vi "Auto_guider.vi"() -> ()   [LabVIEW 2018]
uses:
  Global_Telescopio.vi
panel:
  in  "Case Constant\n(See Context Help) 2":bool
  in  "Case Constant\n(See Context Help)":bool=TRUE
  out "substring 3":string
  out "substring 2":string
  out "concatenated string":string
  out "substring":string
  out "result string":string
  in  "esc_placa":string="0.462"
  out "Serial Settings:Number of Bytes at Serial Port":u32
  in  "guide_esp":string="S"
  in  "guide_cas":string="S"
  in  "guide_str":string="04/10/09  1:18:34\u000013 27 13\u0000-12 45 20\u0000"
  in  "guide_ang":string=" 281.52"
  in  "guide_nor":string="  11.53"
  in  "Tx_sts":u8[](array[numeric])=[22, 2, 1, 0, 83, 0, 0]
  out "rxsts 3":bool
  in  "SYN | ETX":u8[](array[numeric])=[22, 3] format="%02.0f"
  in  "tel_sts2":u8[](array[numeric])=[0, 0, 0] format="%02.0f"
  in  "Tx_ena":u8[](array[numeric])=[22, 2, 1, 0, 72, 0, 0] format="%02.0f"
  out "tel_sts1":bool[](array[boolean])=[TRUE, TRUE, TRUE, TRUE, FALSE, FALSE, TRUE]
  out "guide_dec":dbl format="%07.2g"
  out "guide_dir_ns":string
  out "guide_asc":dbl format="%07.2g"
  out "guide_dir_we":string
  in  "SYN | ACK":u8[](array[numeric])=[22, 6] format="%02.0f"
  out "rxsts":bool
  in  "Tx_nak":u8[](array[numeric])=[22, 21]
  out "Data rx guider":string
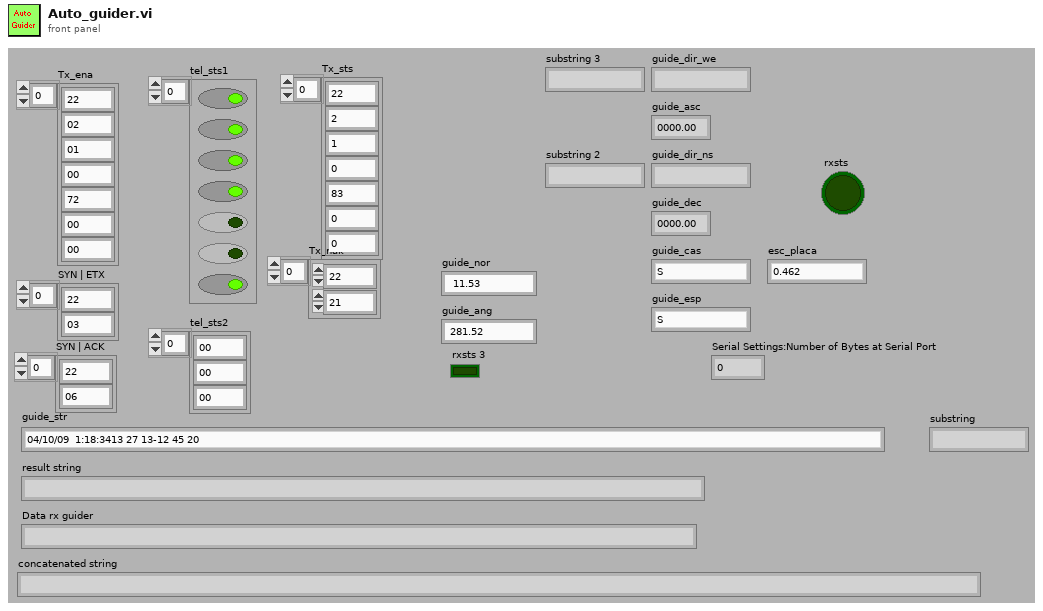
[diagram p1: front panel]
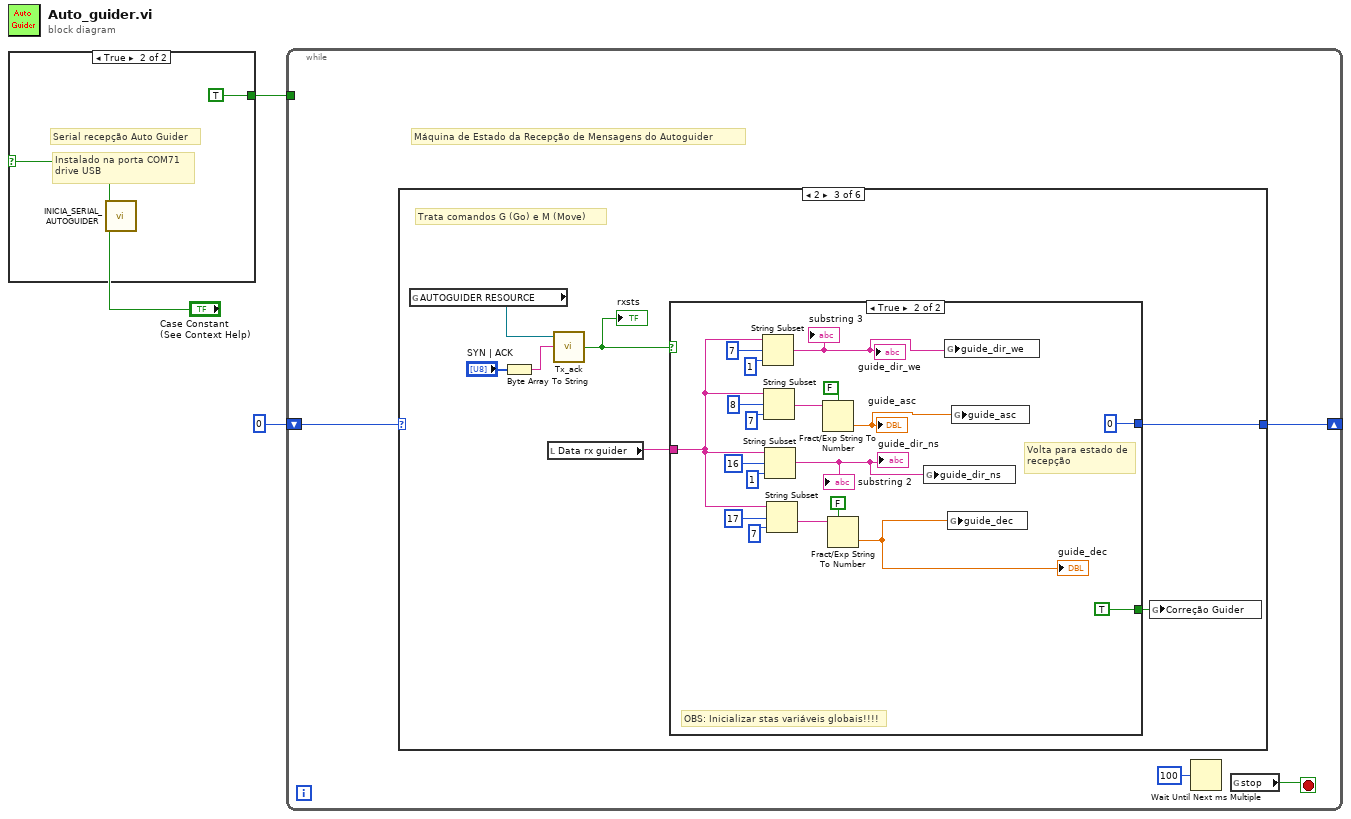
[diagram p0: block diagram]
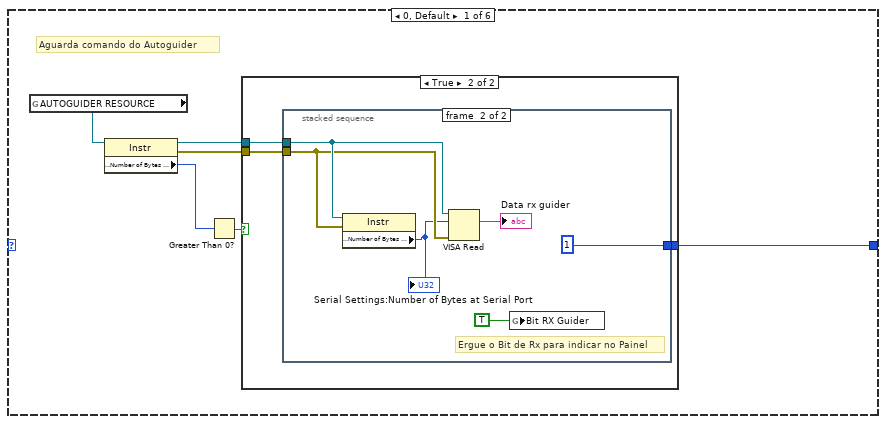
[diagram p3: hidden frame]
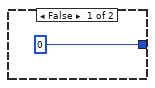
[diagram p4: hidden frame]
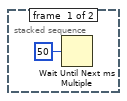
[diagram p5: hidden frame]
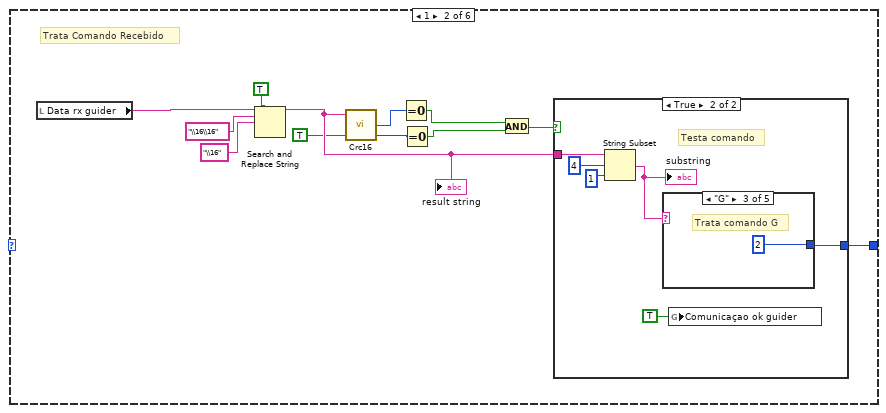
[diagram p6: hidden frame]
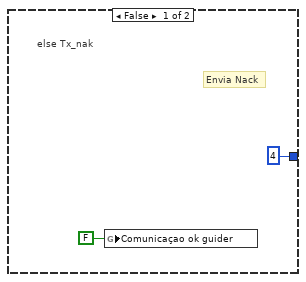
[diagram p7: hidden frame]
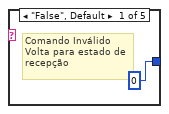
[diagram p8: hidden frame]
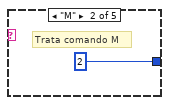
[diagram p9: hidden frame]
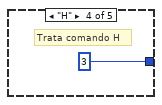
[diagram p10: hidden frame]
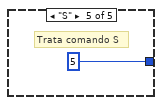
[diagram p11: hidden frame]
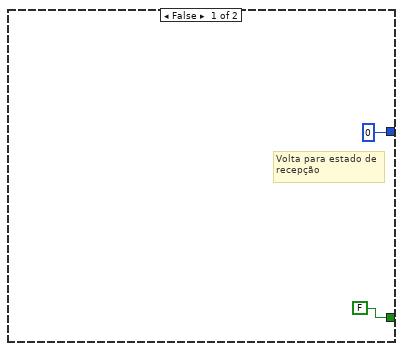
[diagram p12: hidden frame]
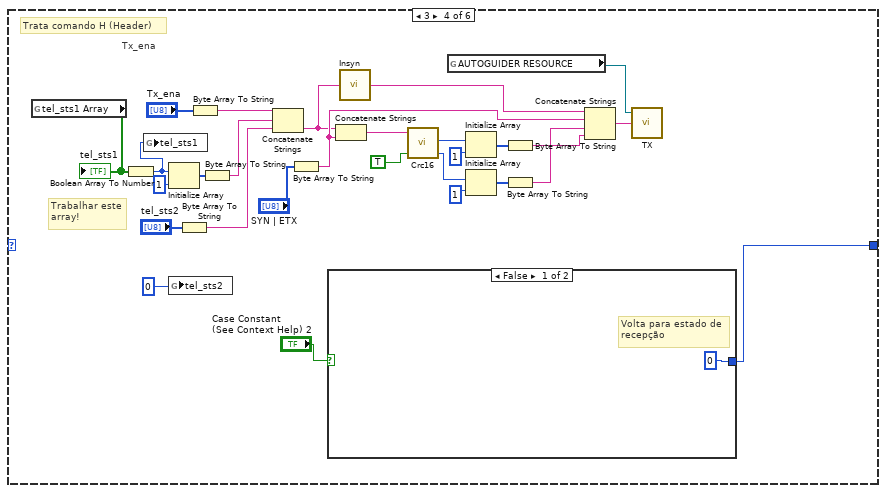
[diagram p13: hidden frame]
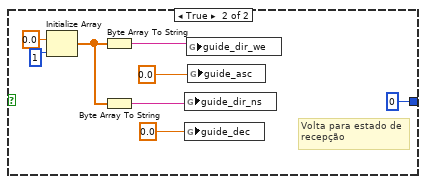
[diagram p14: hidden frame]
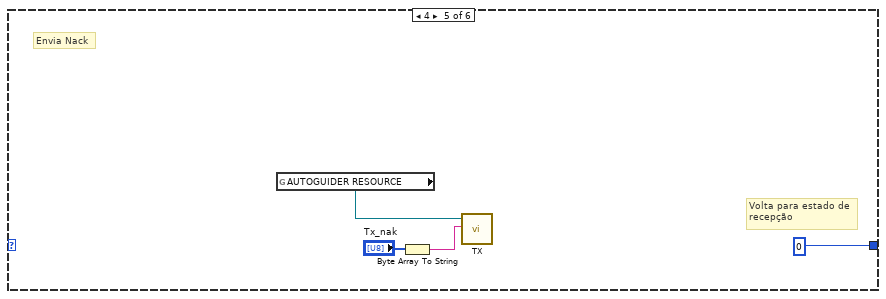
[diagram p15: hidden frame]
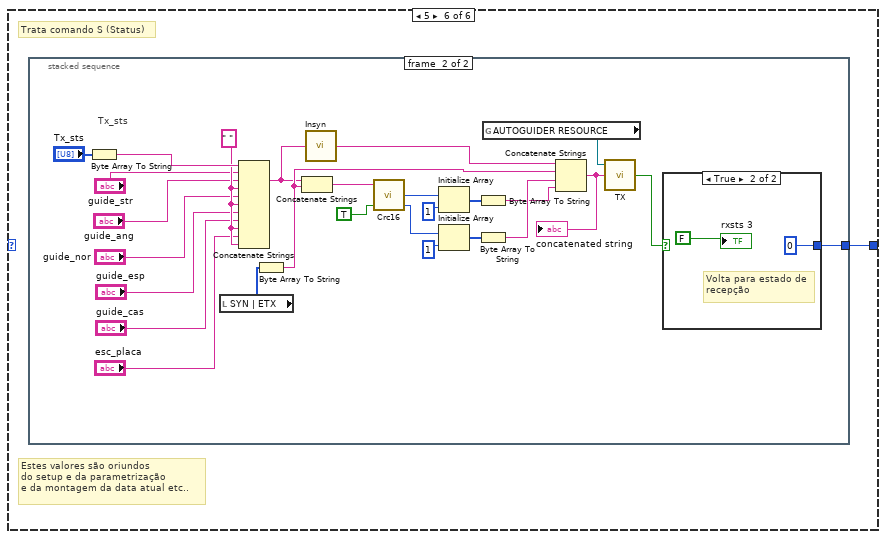
[diagram p16: hidden frame]
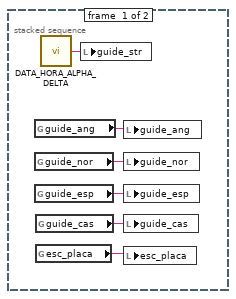
[diagram p17: hidden frame]
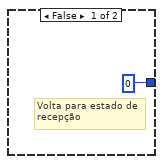
[diagram p18: hidden frame]
diagram:
  n1 = case shown="True" "Case Constant\n(See Context Help)" {
    tunnel: [_ TRUE] -> w1
    frame False {
    }
    frame True {
      # "Instalado na porta COM71\ndrive USB"
      # "Serial recepção Auto Guider"
      n2 = call "INICIA_SERIAL_AUTOGUIDER.vi"() -> ()  [unwired: 6 in, 1 out]
    }
  }
  n3 = while {
    shift-right: [w5] -> _
    shift-left: 0 -> [w6]
    tunnel: w1 -> [_]
    stop <- w8 stop-if-true
    # "Máquina de Estado da Recepção de Mensagens do Autoguider"
    n4 = case shown="2" w6 {
      tunnel: [w9 w37 w52 w83 0 w120] -> w5
      frame 0, Default {
        # "Aguarda comando do Autoguider"
        n5 = global read "Global_Telescopio.vi" "AUTOGUIDER RESOURCE"() -> (w11:refnum<visa-resource-name>)
        n6 = property class="Instr"(reference=w11) -> (reference out=w14:refnum<visa-resource-name>, error out=w13:errorcluster, "Serial Settings:Number of Bytes at Serial Port"=w12:u32)  [unwired: 1 in]
        n7 = Greater Than 0?(x=w12) -> (x > 0?=w10:bool)
        n8 = case shown="True" w10 {
          tunnel: w14 -> [_ w18]
          tunnel: w13 -> [_ w17]
          tunnel: [0 w16] -> w9
          frame False {
          }
          frame True {
            n9 = stacked-sequence {
              tunnel: w18 -> [_ w25]
              tunnel: w17 -> [_ w24]
              tunnel: [_ 1] -> w16
              frame #0 {
                n10 = Wait Until Next ms Multiple(millisecond multiple=u32 50) -> ()  [unwired: 1 out]
              }
              frame #1 {
                # "Ergue o Bit de Rx para indicar no Painel"
                n11 = property class="Instr"(reference=w25, error in=w24) -> ("Serial Settings:Number of Bytes at Serial Port"=w23:u32)  [unwired: 2 out]
                "Serial Settings:Number of Bytes at Serial Port" <- w23
                n12 = VISA Read(VISA resource name=w25, byte count=w23, error in (no error)=w24) -> (read buffer=→"Data rx guider":string)  [unwired: 3 out]
                n13 = global write "Global_Telescopio.vi" "Bit RX Guider"(TRUE) -> ()
              }
            }
          }
        }
      }
      frame 1 {
        # "Trata Comando Recebido"
        n14 = local read "Data rx guider"() -> (w33:string)
        n15 = Search and Replace String(replace all?=TRUE ("replace all? (F)"), input string=w33, search string="\\16\\16", replace string="\\16" ("replace string (\"\")")) -> (result string=w32:string)  [unwired: 4 in, 3 out]
        "result string" <- w32
        n16 = call "Crc16.vi"("Habilita"=TRUE, "tx_rx_buf"=w32) -> ("crc_lo"=w29:u8, "crc_hi"=w30:u8)  [unwired: 1 in, 1 out]
        n17 = Equal To 0?(x=w30) -> (x = 0?=w26:bool)
        n18 = Equal To 0?(x=w29) -> (x = 0?=w27:bool)
        n19 = And(x=w26, y=w27) -> (x .and. y?=w28:bool)
        n20 = case shown="True" w28 {
          tunnel: [4 w45] -> w37
          tunnel: w32 -> [_ w44]
          frame False {
            # "else Tx_nak"
            # "Envia Nack"
            n21 = global write "Global_Telescopio.vi" "Comunicaçao ok guider"(FALSE ("Comunicaçao ok guider")) -> ()
          }
          frame True {
            # "Testa comando"
            n22 = String Subset(string=w44, offset (0)=4, length (rest)=1 ("length (rest)")) -> (substring=w41:string)
            "substring" <- w41
            n23 = case shown="\"G\"" w41 {
              tunnel: [0 2 2 3 5] -> w45
              frame "False", Default {
                # "Comando Inválido\nVolta para estado de\nrecepção"
              }
              frame "M" {
                # "Trata comando M"
              }
              frame "G" {
                # "Trata comando G"
              }
              frame "H" {
                # "Trata comando H"
              }
              frame "S" {
                # "Trata comando S"
              }
            }
            n24 = global write "Global_Telescopio.vi" "Comunicaçao ok guider"(TRUE ("Comunicaçao ok guider")) -> ()
          }
        }
      }
      frame 2 {
        # "Trata comandos G (Go) e M (Move)"
        n25 = global read "Global_Telescopio.vi" "AUTOGUIDER RESOURCE"() -> (w54:refnum<visa-resource-name>)
        n26 = Byte Array To String(unsigned byte array="SYN | ACK") -> (string=w55:string)
        n27 = local read "Data rx guider"() -> (w53:string)
        n28 = call "Tx_ack.vi"("txbuf"=w55, "VISA resource name"=w54) -> ("envio OK"=w57:bool)  [unwired: 1 in, 2 out]
        "rxsts" <- w57
        n29 = case shown="True" w57 {
          tunnel: w53 -> [_ w74]
          tunnel: [0 0] -> w52
          tunnel: [FALSE ("Correção Guider") TRUE ("Correção Guider")] -> w51
          frame False {
            # "Volta para estado de\nrecepção"
          }
          frame True {
            # "OBS: Inicializar stas variáveis globais!!!!"
            # "Volta para estado de\nrecepção"
            n30 = String Subset(string=w74, offset (0)=7, length (rest)=1 ("length (rest)")) -> (substring=w64:string)
            "guide_dir_we" <- w64
            "substring 3" <- w64
            n31 = String Subset(string=w74, offset (0)=8, length (rest)=7 ("length (rest)")) -> (substring=w68:string)
            n32 = String Subset(string=w74, offset (0)=16, length (rest)=1 ("length (rest)")) -> (substring=w62:string)
            "guide_dir_ns" <- w62
            "substring 2" <- w62
            n33 = String Subset(string=w74, offset (0)=17, length (rest)=7 ("length (rest)")) -> (substring=w67:string)
            n34 = Fract/Exp String To Number(use system decimal point (T)=FALSE, string=w68) -> (number=w63:dbl)  [unwired: 2 in, 1 out]
            "guide_asc" <- w63
            n35 = Fract/Exp String To Number(use system decimal point (T)=FALSE, string=w67) -> (number=w61:dbl)  [unwired: 2 in, 1 out]
            "guide_dec" <- w61
            n36 = global write "Global_Telescopio.vi" "guide_dir_ns"(w62) -> ()
            n37 = global write "Global_Telescopio.vi" "guide_dir_we"(w64) -> ()
            n38 = global write "Global_Telescopio.vi" "guide_dec"(w61) -> ()
            n39 = global write "Global_Telescopio.vi" "guide_asc"(w63) -> ()
          }
        }
        n40 = global write "Global_Telescopio.vi" "Correção Guider"(w51) -> ()
      }
      frame 3 {
        # "Trabalhar este\narray!"
        # "Tx_ena"
        # "Trata comando H (Header)"
        n41 = global read "Global_Telescopio.vi" "tel_sts1 Array"() -> (w80:bool[])
        "tel_sts1" <- w80
        n42 = Boolean Array To Number(Boolean array=w80) -> (number=w81:u32)
        n43 = global write "Global_Telescopio.vi" "tel_sts1"(w81) -> ()
        n44 = Initialize Array(w81, 1 ("dimension size")) -> (w91:u32[])
        n45 = global write "Global_Telescopio.vi" "tel_sts2"(0) -> ()
        n46 = Byte Array To String(unsigned byte array="tel_sts2") -> (string=w104:string)
        n47 = Byte Array To String(unsigned byte array="Tx_ena") -> (string=w102:string)
        n48 = Byte Array To String(unsigned byte array=w91) -> (string=w92:string)
        n49 = Concatenate Strings(w102, w92, w104) -> (w87:string)
        n50 = Byte Array To String(unsigned byte array="SYN | ETX") -> (string=w106:string)
        n51 = case shown="False" "Case Constant\n(See Context Help) 2" {
          tunnel: [0 0] -> w83
          frame False {
            # "Volta para estado de\nrecepção"
          }
          frame True {
            # "Volta para estado de\nrecepção"
            n52 = Initialize Array(0.0 ("element"), 1 ("dimension size")) -> (w112:dbl[])
            n53 = Byte Array To String(unsigned byte array=w112) -> (string=w111:string)
            n54 = Byte Array To String(unsigned byte array=w112) -> (string=w109:string)
            n55 = global write "Global_Telescopio.vi" "guide_dir_ns"(w109) -> ()
            n56 = global write "Global_Telescopio.vi" "guide_dec"(0.0 ("guide_dec")) -> ()
            n57 = global write "Global_Telescopio.vi" "guide_dir_we"(w111) -> ()
            n58 = global write "Global_Telescopio.vi" "guide_asc"(0.0 ("guide_asc")) -> ()
          }
        }
        n59 = Concatenate Strings(w87, w106) -> (w86:string)
        n60 = call "Insyn.vi"("txbuf"=w87) -> ("txbuf OUT"=w88:string)
        n61 = call "Crc16.vi"("Habilita"=TRUE, "tx_rx_buf"=w86) -> ("crc_lo"=w96:u8, "crc_hi"=w94:u8)  [unwired: 1 in, 1 out]
        n62 = global read "Global_Telescopio.vi" "AUTOGUIDER RESOURCE"() -> (w84:refnum<visa-resource-name>)
        n63 = Initialize Array(w94, 1 ("dimension size")) -> (w98:u8[])
        n64 = Initialize Array(w96, 1 ("dimension size")) -> (w97:u8[])
        n65 = Byte Array To String(unsigned byte array=w98) -> (string=w99:string)
        n66 = Byte Array To String(unsigned byte array=w97) -> (string=w100:string)
        n67 = Concatenate Strings(w88, w106, w100, w99) -> (w89:string)
        n68 = call "TX.vi"("tx_buf"=w89, "VISA resource name"=w84) -> ()  [unwired: 1 in, 3 out]
      }
      frame 4 {
        # "Volta para estado de\nrecepção"
        # "Envia Nack"
        n69 = global read "Global_Telescopio.vi" "AUTOGUIDER RESOURCE"() -> (w116:refnum<visa-resource-name>)
        n70 = Byte Array To String(unsigned byte array="Tx_nak") -> (string=w117:string)
        n71 = call "TX.vi"("tx_buf"=w117, "VISA resource name"=w116) -> ()  [unwired: 1 in, 3 out]
      }
      frame 5 {
        # "Estes valores são oriundos\ndo setup e da parametrização\ne da montagem da data atual etc.."
        # "Trata comando S (Status)"
        n72 = stacked-sequence {
          tunnel: [_ w134] -> w120
          frame #0 {
            n73 = global read "Global_Telescopio.vi" "guide_ang"() -> (w125:string)
            n74 = global read "Global_Telescopio.vi" "guide_nor"() -> (w124:string)
            n75 = global read "Global_Telescopio.vi" "guide_esp"() -> (w123:string)
            n76 = global read "Global_Telescopio.vi" "guide_cas"() -> (w122:string)
            n77 = global read "Global_Telescopio.vi" "esc_placa"() -> (w121:string)
            n78 = call "DATA_HORA_ALPHA_DELTA.vi"() -> ("SAIDA"=w126:string)  [unwired: 2 in]
            n79 = local write "guide_str"(w126) -> ()
            n80 = local write "guide_ang"(w125) -> ()
            n81 = local write "guide_nor"(w124) -> ()
            n82 = local write "guide_esp"(w123) -> ()
            n83 = local write "guide_cas"(w122) -> ()
            n84 = local write "esc_placa"(w121) -> ()
          }
          frame #1 {
            w142 = " " ("string")
            # "Tx_sts"
            n85 = Byte Array To String(unsigned byte array="Tx_sts") -> (string=w153:string)
            n86 = local read "SYN | ETX"() -> (w128:u8[])
            n87 = Concatenate Strings(w153, "guide_str", "guide_ang", w142, "guide_nor", w142, "guide_esp", "guide_cas", w142, "esc_placa", w142) -> (w139:string)
            n88 = Byte Array To String(unsigned byte array=w128) -> (string=w151:string)
            n89 = Concatenate Strings(w139, w151) -> (w138:string)
            n90 = call "Insyn.vi"("txbuf"=w139) -> ("txbuf OUT"=w140:string)
            n91 = call "Crc16.vi"("Habilita"=TRUE, "tx_rx_buf"=w138) -> ("crc_lo"=w147:u8, "crc_hi"=w148:u8)  [unwired: 1 in, 1 out]
            n92 = Initialize Array(w148, 1 ("dimension size")) -> (w146:u8[])
            n93 = Initialize Array(w147, 1 ("dimension size")) -> (w145:u8[])
            n94 = Byte Array To String(unsigned byte array=w146) -> (string=w149:string)
            n95 = Byte Array To String(unsigned byte array=w145) -> (string=w150:string)
            n96 = global read "Global_Telescopio.vi" "AUTOGUIDER RESOURCE"() -> (w136:refnum<visa-resource-name>)
            n97 = Concatenate Strings(w140, w151, w150, w149) -> (w141:string)
            "concatenated string" <- w141
            n98 = call "TX.vi"("tx_buf"=w141, "VISA resource name"=w136) -> ("envio OK"=w135:bool)  [unwired: 1 in, 2 out]
            n99 = case shown="True" w135 {
              tunnel: [0 0] -> w134
              frame False {
                # "Volta para estado de\nrecepção"
              }
              frame True {
                # "Volta para estado de\nrecepção"
                "rxsts 3" <- FALSE ("rxsts")
              }
            }
          }
        }
      }
    }
    n100 = Wait Until Next ms Multiple(millisecond multiple=u32 100) -> ()  [unwired: 1 out]
    n101 = global read "Global_Telescopio.vi" "stop"() -> (w8:bool)
  }
